vi "reset.vi"(8 "error in (no error)":errorcluster, 11 "ImageAssemblerRK110612Spiral in":refnum<class "ImageAssemblerRK110612Spiral.lvclass">) -> (0 "error out":errorcluster, 3 "ImageAssemblerRK110612Spiral out":refnum<class "ImageAssemblerRK110612Spiral.lvclass">)   [LabVIEW 2010, in "ImageAssemblerRK110612Spiral.lvclass"]
uses:
  ImageAssemblerRK110612Spiral.lvclass
  ImageAssemblerDL090211Scaffold/ImageAssemblerDL090211Scaffold/ImageAssemblerDL090211Scaffold.lvclass
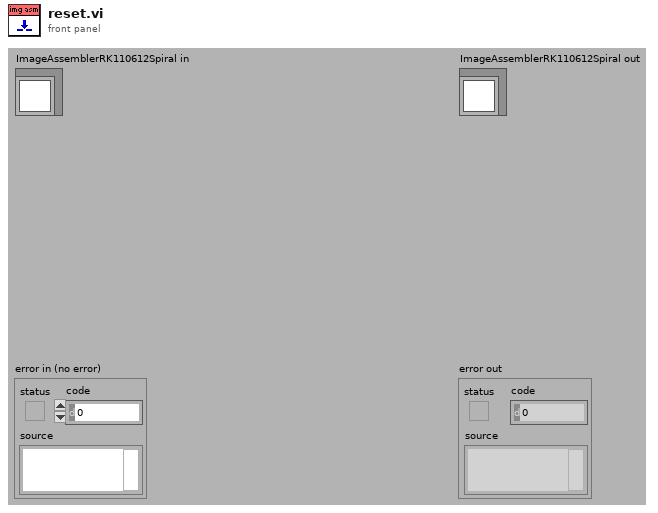
[diagram p1: front panel]
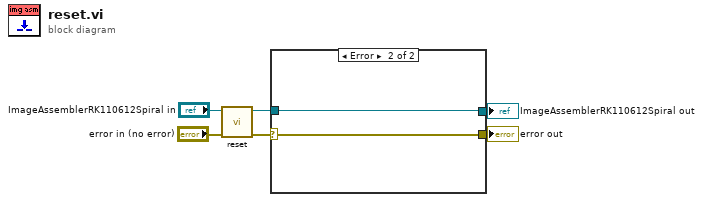
[diagram p0: block diagram]
diagram:
  n1 = call-parent "reset.vi"("error in (no error)"="error in (no error)", "DL090211ImageAssemblerScaffold in"="ImageAssemblerRK110612Spiral in") -> ("error out"=w4:errorcluster, "DL090211ImageAssemblerScaffold out"=w3:refnum<class "ImageAssemblerRK110612Spiral.lvclass">)  [unwired: 8 in]
  n2 = case shown="Error" w4 {
    selector: w4 -> [w7 w9]
    tunnel: [w8 w10] -> w2
    tunnel: w3 -> [w8 w10]
    tunnel: [w7 w9] -> w1
    frame No Error {
    }
    frame Error {
    }
  }
  "error out" <- w1
  "ImageAssemblerRK110612Spiral out" <- w2
